vi "confirm modules.vi"(9 "inactive modules IN":string[](array[string]), 10 "optional modules IN":string[](array[string]), 11 "required modules IN":string[](array[string])) -> (1 "inactive modules out":string[](array[string]), 2 "optional modules out":string[](array[string]), 3 "required modules out":string[](array[string]))   [LabVIEW 2017]
doc: "SciScan 1.2 160622"
panel:
  in  "inactive modules":i32(listbox)
  in  "optional modules":i32(listbox)
  in  "stop":bool
  in  "required modules":i32(listbox)
  # "Inactive modules"
  # "Active modules"
  # "Drag & drop\nmodules to activate\nor deactivate them"
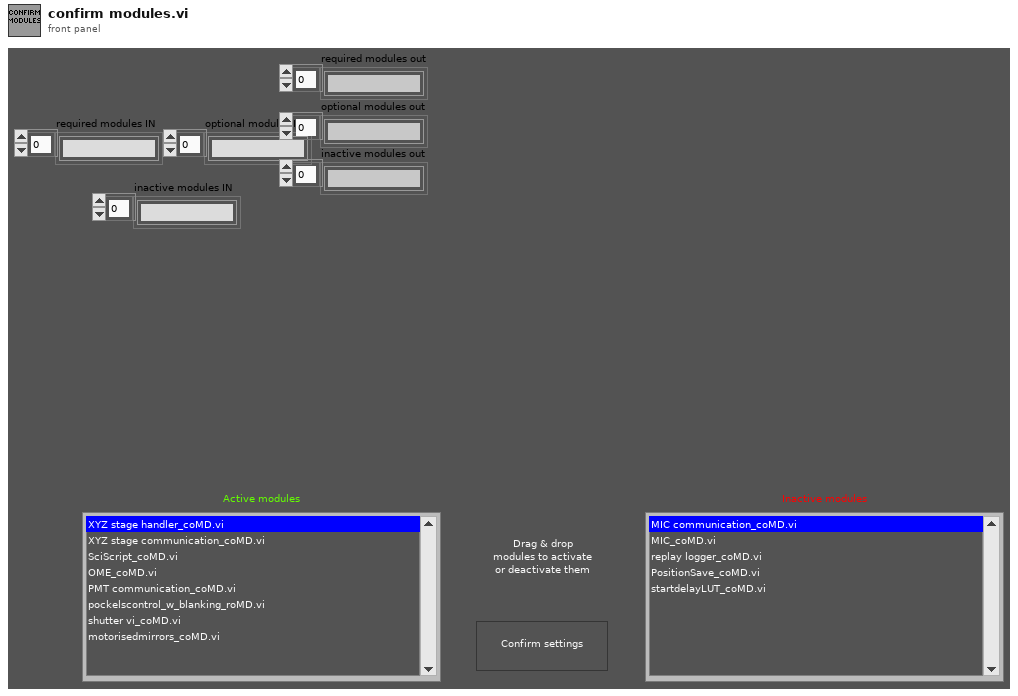
[diagram p1: front panel]
types:
  T1 = typedef "LVBoundsTypeDef.ctl" = cluster{"Width":u32, "Height":u32}
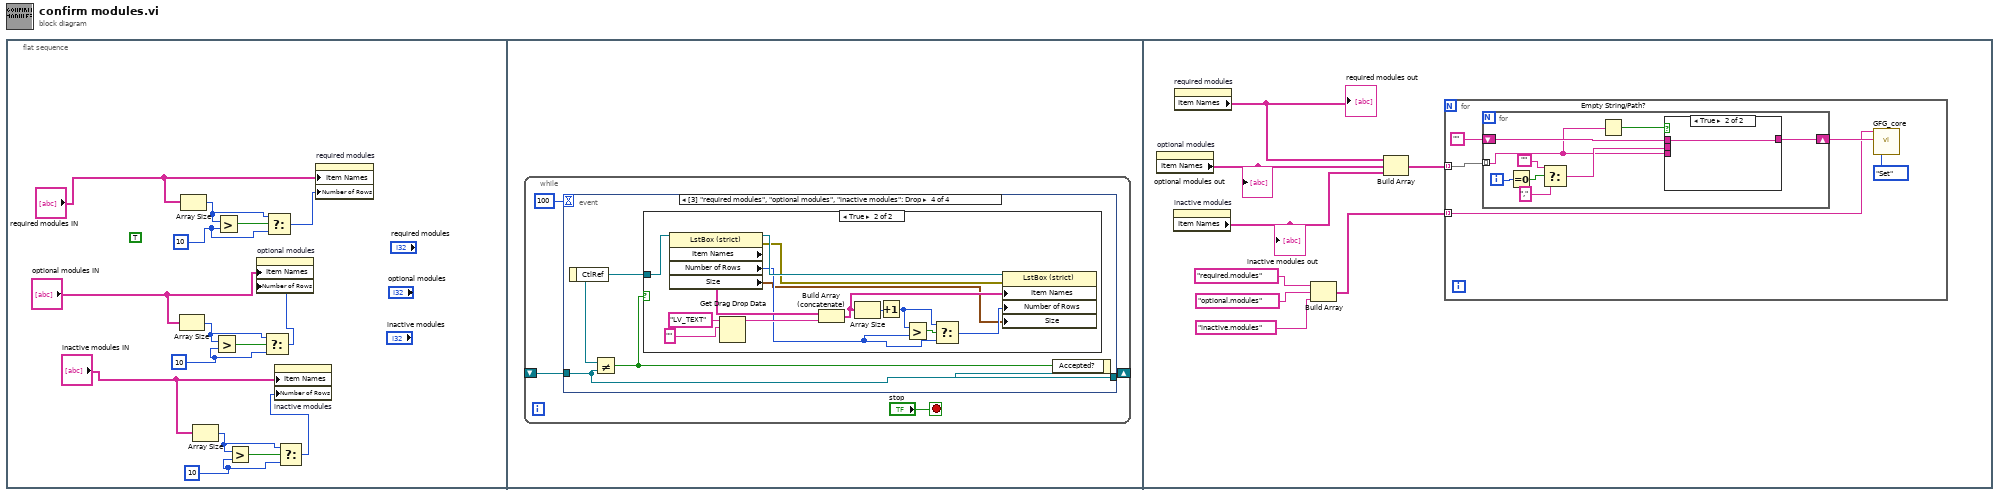
[diagram p0: block diagram]
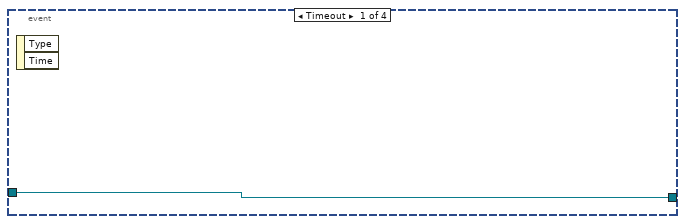
[diagram p2: hidden frame]
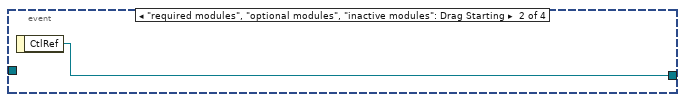
[diagram p3: hidden frame]
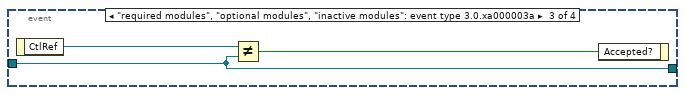
[diagram p4: hidden frame]
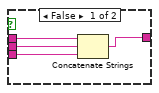
[diagram p6: hidden frame]
diagram:
  n1 = flat-sequence {
    frame #0 {
      w7 = 10 ("y")
      w9 = 10 ("y")
      w12 = 10 ("y")
      (unwired) TRUE ("Drag/Drop:Allow Drag and Drop Outside Control")
      n2 = Array Size(array="optional modules IN") -> (size(s)=w5:i32)
      n3 = Array Size(array="required modules IN") -> (size(s)=w13:i32)
      n4 = Array Size(array="inactive modules IN") -> (size(s)=w11:i32)
      n5 = Greater?(x=w5, y=w7) -> (0:w6:bool)
      n6 = Greater?(x=w13, y=w12) -> (0:w14:bool)
      n7 = Greater?(x=w11, y=w9) -> (0:w10:bool)
      n8 = Select(t=w5, s=w6, f=w7) -> (s? t:f=w3:i32)
      n9 = property on="optional modules" class="LstBox (strict)"("Item Names"="optional modules IN", "Number of Rows"=w3) -> ()  [unwired: 2 in, 2 out]
      n10 = Select(t=w13, s=w14, f=w12) -> (s? t:f=w2:i32)
      n11 = Select(t=w11, s=w10, f=w9) -> (s? t:f=w8:i32)
      n12 = property on="inactive modules" class="LstBox (strict)"("Item Names"="inactive modules IN", "Number of Rows"=w8) -> ()  [unwired: 2 in, 2 out]
      n13 = property on="required modules" class="LstBox (strict)"("Item Names"="required modules IN", "Number of Rows"=w2) -> ()  [unwired: 2 in, 2 out]
    }
    frame #1 {
      n14 = while {
        shift-right: [w17] -> _
        shift-left: _ -> [w16]
        stop <- "stop" stop-if-true
        n15 = event shown="[3] \"required modules\", \"optional modules\", \"inactive modules\": Drop" {
          selector: _ -> [_ _ _ _]
          dyn-events: _ -> [_ _ _ _]
          timeout: 100 -> [_ _ _ _]
          tunnel: [w20 w21 w24 w27] -> w17
          tunnel: w16 -> [w20 _ w24 w27]
          event Timeout {
            n16 = event-data() -> ()  [unwired: 1 in, 2 out]
          }
          event "required modules", "optional modules", "inactive modules": Drag Starting {
            n17 = event-data() -> ("CtlRef"=w21:refnum<vi>)  [unwired: 1 in]
          }
          event "required modules", "optional modules", "inactive modules": event type 3.0.xa000003a {
            n18 = event-data() -> ("CtlRef"=w22:refnum<vi>)  [unwired: 1 in]
            n19 = Not Equal?(x=w22, y=w24) -> (x != y?=w23:bool)
            n20 = event-data("Accepted?"=w23) -> ()  [unwired: 1 in, 1 out]
          }
          event "required modules", "optional modules", "inactive modules": Drop {
            n21 = event-data() -> ("CtlRef"=w25:refnum<vi>)  [unwired: 1 in]
            n22 = Not Equal?(x=w25, y=w27) -> (x != y?=w26:bool)
            n23 = case shown="True" w26 {
              tunnel: w25 -> [_ w40]
              frame False {
              }
              frame True {
                n24 = property class="LstBox (strict)"(reference=w40) -> (reference out=w37:refnum<vi>, error out=w36:errorcluster, "Item Names"=w39:string[], "Number of Rows"=w30:u32, "Size"=w28:T1)  [unwired: 1 in]
                n25 = Get Drag Drop Data(8:"" ("type"), 9:"LV_TEXT" ("data name")) -> (3:w38:string)  [unwired: 1 in, 1 out]
                n26 = Build Array (concatenate)(w39, w38) -> (w34:string[])
                n27 = Array Size(array=w34) -> (size(s)=w32:i32)
                n28 = Increment(x=w32) -> (x+1=w29:i32)
                n29 = Greater?(x=w29, y=w30) -> (0:w33:bool)
                n30 = Select(t=w29, s=w33, f=w30) -> (s? t:f=w31:u32)
                n31 = property class="LstBox (strict)"(reference=w37, error in=w36, "Item Names"=w34, "Number of Rows"=w31, "Size"=w28) -> ()  [unwired: 2 out]
              }
            }
            n32 = event-data("Accepted?"=w26) -> ()  [unwired: 1 in, 1 out]
          }
        }
      }
    }
    frame #2 {
      n33 = property on="optional modules" class="LstBox (strict)"() -> ("Item Names"=w48:string[])  [unwired: 2 in, 2 out]
      "optional modules out" <- w48
      n34 = property on="inactive modules" class="LstBox (strict)"() -> ("Item Names"=w47:string[])  [unwired: 2 in, 2 out]
      "inactive modules out" <- w47
      n35 = property on="required modules" class="LstBox (strict)"() -> ("Item Names"=w49:string[])  [unwired: 2 in, 2 out]
      "required modules out" <- w49
      n36 = Build Array("required.modules", "optional.modules", "inactive.modules") -> (w42:string[])
      n37 = Build Array(w49, w48, w47) -> (w46:string[][])
      n38 = for {
        tunnel: w46 -> [w53] mode=indexing
        tunnel: w42 -> [w51] mode=indexing
        n39 = for {
          tunnel: w53 -> [w56] mode=indexing
          shift-right: [w57] -> w52
          shift-left: "" -> [w59]
          i -> [w63]
          n40 = Equal To 0?(x=w63) -> (x = 0?=w62:bool)
          n41 = Select(t="", s=w62, f=",") -> (s? t:f=w60:string)
          n42 = Empty String/Path?(string/path=w56) -> (empty?=w55:bool)
          n43 = case shown="True" w55 {
            tunnel: w60 -> [w67 _]
            tunnel: w59 -> [w66 w68]
            tunnel: [w65 w68] -> w57
            tunnel: w56 -> [w64 _]
            frame False {
              n44 = Concatenate Strings(w66, w67, w64) -> (w65:string)
            }
            frame True {
            }
          }
        }
        n45 = call "GFG_core.vi"("Variable Name in"=w51, "Variant in"=w52, "Action"=enum16{"Init", "Set", "Get", "Clear"}."Set") -> ()  [unwired: 10 in, 7 out]
      }
    }
  }
